vi "Find frequency.vi"() -> ()   [LabVIEW 2017]
uses:
  <vilib>/DAQmx/create/channels.llb/DAQmx Create Channel (AI-Voltage-Basic).vi
  <vilib>/measure/NI_MAPro.lvlib
  <vilib>/measure/madcrms.llb/Basic Averaged DC-RMS for 1 Chan.vi
  <vilib>/DAQmx/configure/timing.llb/DAQmx Timing (Sample Clock).vi
  <vilib>/DAQmx/read.llb/DAQmx Read (Analog 2D DBL NChan NSamp).vi
panel:
  in  "Delay, ms":u32=300
  out "Result":dbl
  in  "btnStartStop":bool=TRUE caption="stop"
  out "CurrentFrequency":dbl
  out "CurrentPoint":i32
  out "XY Graph":cluster{dbl[], dbl[]}[](graph)
  in  "Maximum Value":dbl=10.0 format="%0.2f"
  in  "Minimum Value":dbl=-10.0 format="%0.2f"
  in  "Rate":dbl=1000.0 caption="Sample Rate (Hz)" format="%0.2f"
  in  "Samples per Channel":i32=1000
  in  "Physical Channel":tag="Dev2/ai0:1"
  in  "btnStartStopScanning":bool=TRUE caption="stop"
  in  "btnQuit":bool caption="stop"
  out "FrequencyPoints":i32=1000 caption="Frequency points"
  in  "FrequencyStep":dbl=1000.0 caption="Frequency step, Hz"
  in  "EndFrequency":dbl=10000.0 caption="End frequency, Hz" format="%.2p"
  in  "resource name":refnum<k15>="test"
  in  "start phase":dbl format="%.3f"
  in  "StartFrequency":dbl=1000.0 caption="Start frequency, Hz" format="%.2p"
  in  "dc offset":dbl=0.5 format="%.3f"
  in  "Amplitude":dbl=1.0 format="%.3f"
  in  "channel name (\"1\")":string="1"
  in  "WaveformType":i32(ring)=1 items=["Sine"=1, "Square"=2, "Ramp Up"=4, "Triangle"=3, "DC "=6, "Noise"=1001, "Pulse"=1002, "Ramp Down"=5, "Ramp"=1004]
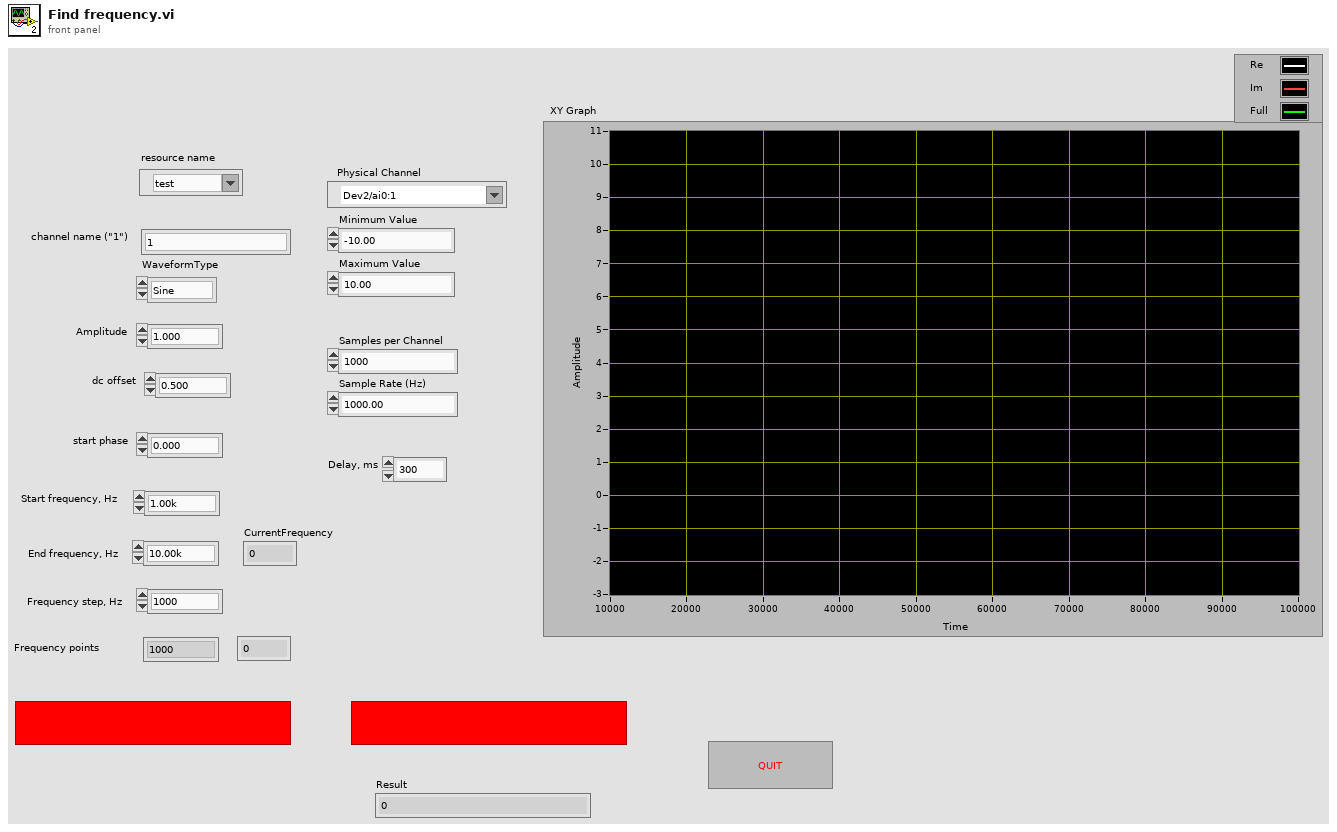
[diagram p1: front panel]
types:
  T1 = enum16{"Rectangular (none)", "Hanning", "Low side lobe"}
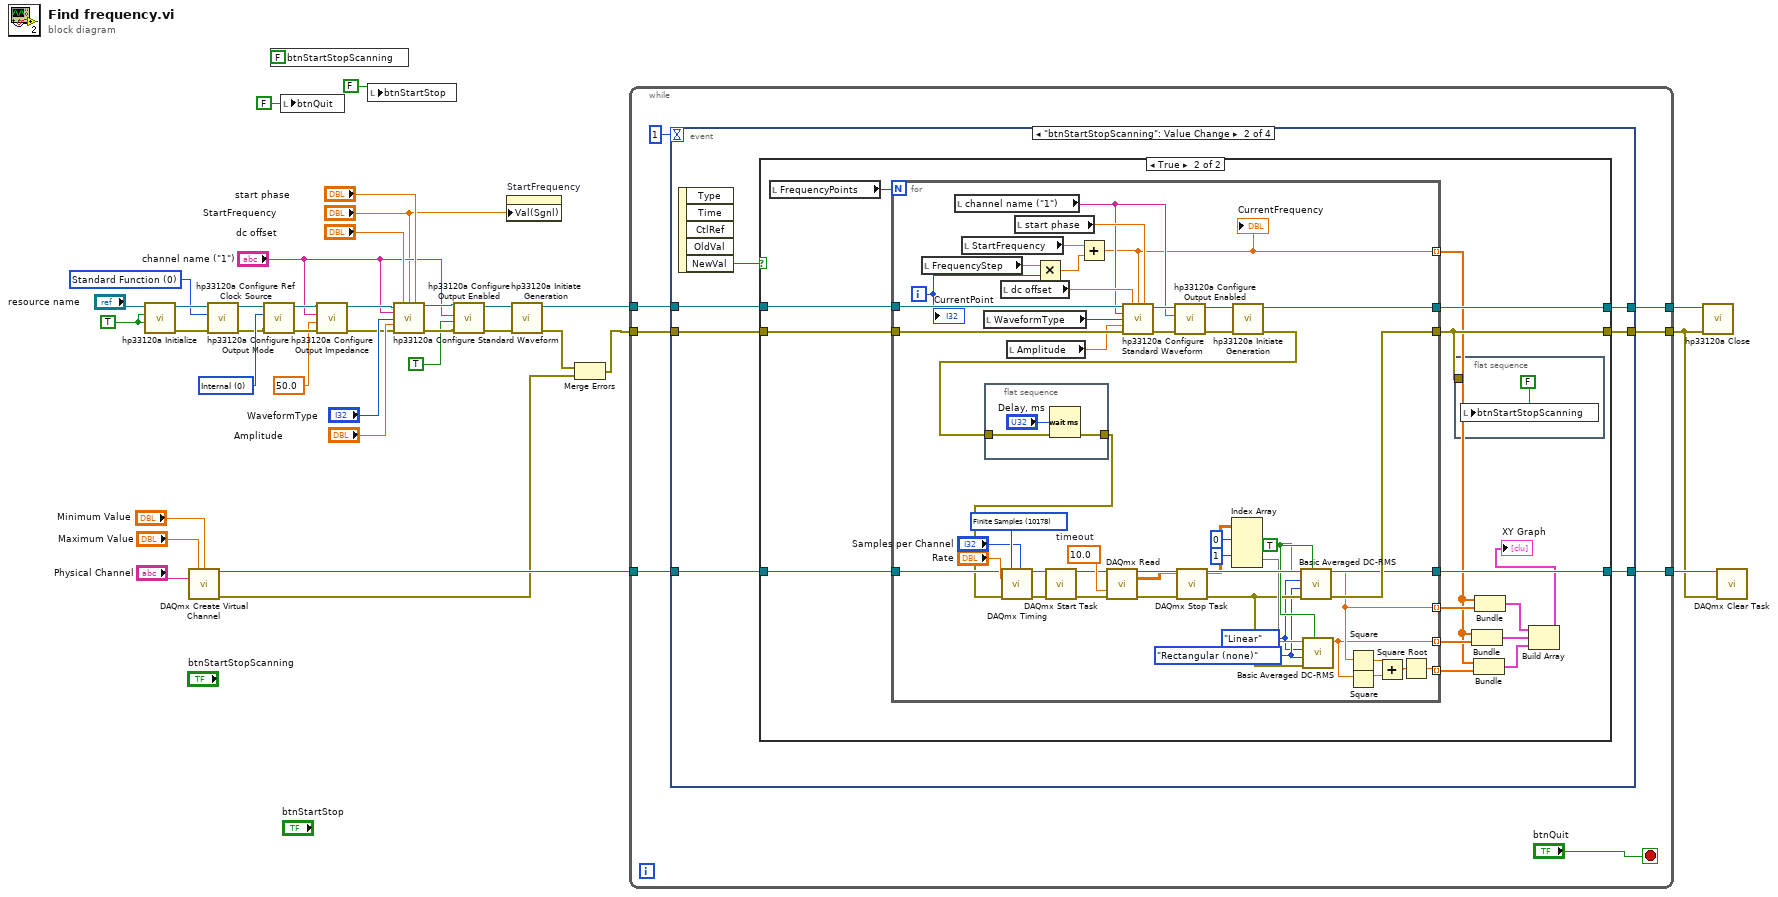
[diagram p0: block diagram]
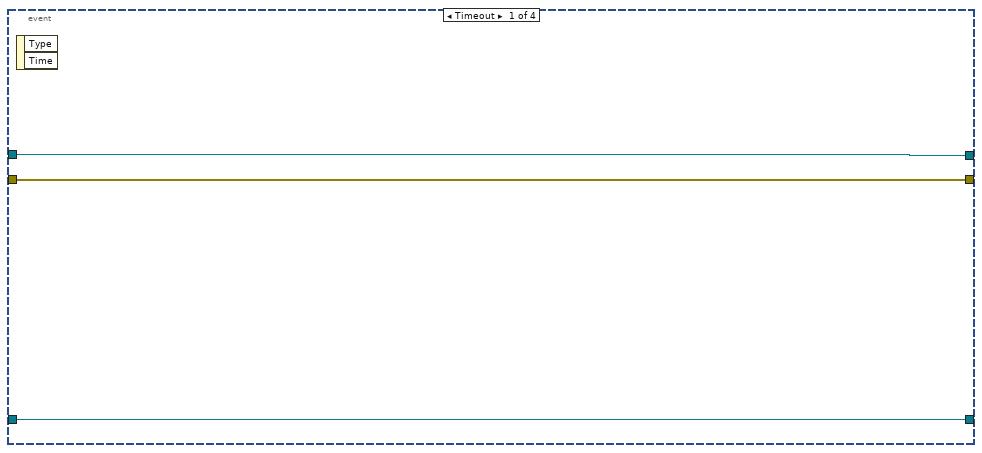
[diagram p2: hidden frame]
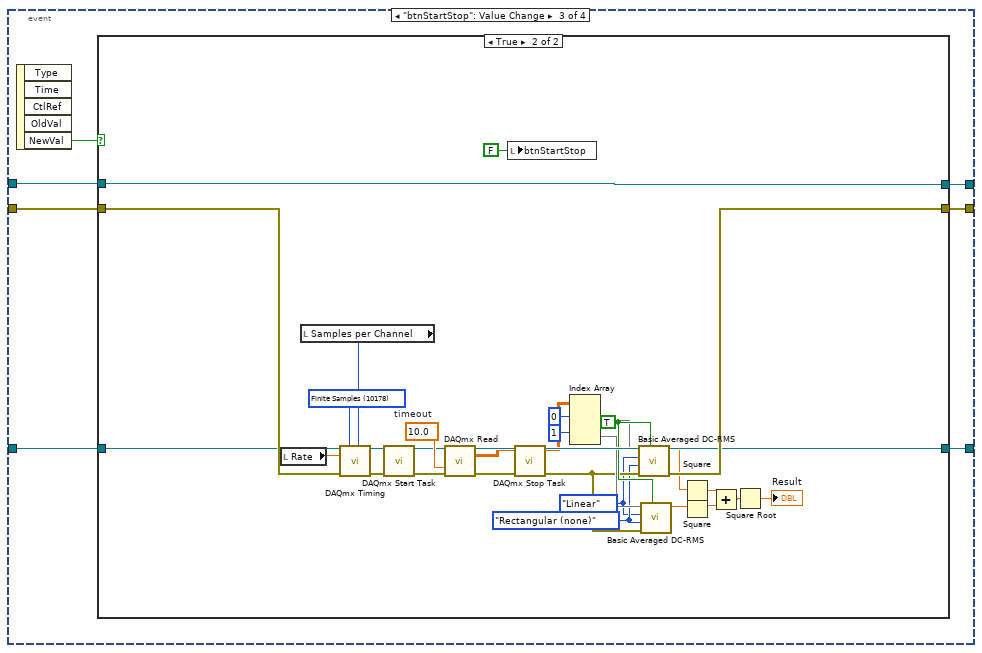
[diagram p4: hidden frame]
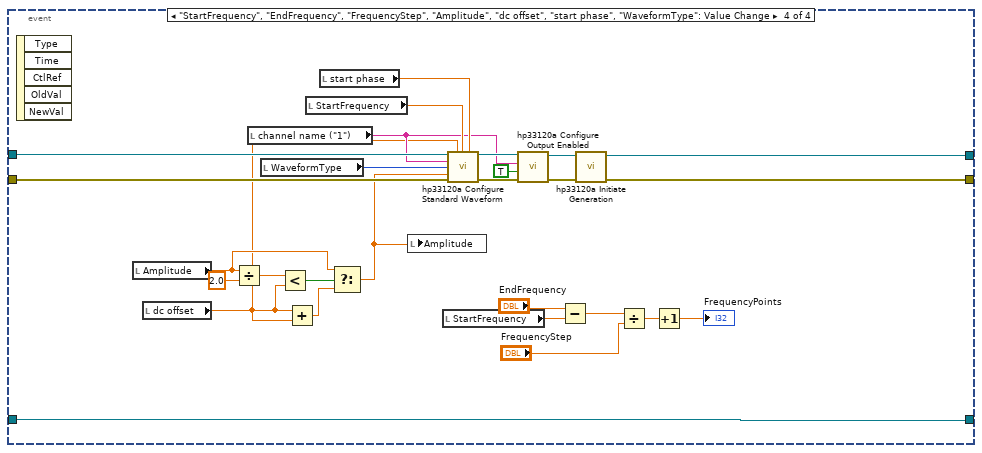
[diagram p6: hidden frame]
diagram:
  w33 = 0 items=["Internal"=0, "External"=1, "RTSI Clock"=101] ("reference clock source (Internal)")
  w34 = 0 items=["Standard Function", "Arbitrary Waveform", "Arbitrary Sequence"] ("output mode (Standard Function)")
  w37 = TRUE ("id query")
  n1 = call <instrlib>:"hp33120a Initialize.vi"("reset device (Yes)"=w37, "id query (Yes)"=w37, "resource name"="resource name") -> ("error out"=w35:errorcluster, "instrument handle out"=w36:refnum<k15>)  [unwired: 1 in, 6 out]
  n2 = call-poly <vilib>:"DAQmx Create Virtual Channel.vi"("maximum value"="Maximum Value", "minimum value"="Minimum Value", "physical channels"="Physical Channel") -> ("task out"=w4:refnum<k21>, "error out"=w3:errorcluster)  [unwired: 11 in]
  n3 = call <instrlib>:"hp33120a Configure Output Mode.vi"("error in (no error)"=w35, "output mode (Standard Function)"=w34, "instrument handle"=w36) -> ("error out"=w29:errorcluster, "instrument handle out"=w30:refnum<k15>)  [unwired: 7 out]
  n4 = call <instrlib>:"hp33120a Configure Ref Clock Source.vi"("error in (no error)"=w29, "reference clock source (Internal)"=w33, "instrument handle"=w30) -> ("error out"=w38:errorcluster, "instrument handle out"=w28:refnum<k15>)  [unwired: 7 out]
  n5 = local write "btnStartStopScanning"(FALSE ("btnStartStop")) -> ()
  n6 = local write "btnQuit"(FALSE ("btnQuit")) -> ()
  n7 = call <instrlib>:"hp33120a Configure Output Impedance.vi"("error in (no error)"=w38, "impedance (50.0)"=50.0 ("impedance (50 Ohms)"), "channel name (\"1\")"="channel name (\"1\")", "instrument handle"=w28) -> ("error out"=w20:errorcluster, "instrument handle out"=w21:refnum<k15>)  [unwired: 6 out]
  n8 = local write "btnStartStop"(FALSE ("btnStartStop")) -> ()
  n9 = call <instrlib>:"hp33120a Configure Standard Waveform.vi"("instrument handle"=w21, "dc offset (0.00)"="dc offset", "frequency (1000.0)"="StartFrequency", "start phase (0.00)"="start phase", "channel name (\"1\")"="channel name (\"1\")", "waveform (Sine)"="WaveformType", "amplitude (0.10)"="Amplitude", "error in (no error)"=w20) -> ("instrument handle out"=w19:refnum<k15>, "error out"=w18:errorcluster)  [unwired: 6 out]
  n10 = call <instrlib>:"hp33120a Configure Output Enabled.vi"("error in (no error)"=w18, "channel enabled (True)"=TRUE, "channel name (\"1\")"="channel name (\"1\")", "instrument handle"=w19) -> ("error out"=w16:errorcluster, "instrument handle out"=w17:refnum<k15>)  [unwired: 6 out]
  n11 = property on="StartFrequency" class="DigNum (strict)"("Val(Sgnl)"="StartFrequency") -> ()  [unwired: 2 in, 2 out]
  n12 = call <instrlib>:"hp33120a Initiate Generation.vi"("error in (no error)"=w16, "instrument handle"=w17) -> ("error out"=w7:errorcluster, "instrument handle out"=w23:refnum<k15>)  [unwired: 8 out]
  n13 = Merge Errors(w7, w3) -> (w6:errorcluster)
  n14 = while {
    tunnel: w23 -> [w46]
    tunnel: w6 -> [w45]
    tunnel: [w44] -> w22
    tunnel: [w43] -> w5
    tunnel: w4 -> [w41]
    tunnel: [w40] -> w8
    stop <- "btnQuit" stop-if-true
    n15 = event shown="[1] \"btnStartStopScanning\": Value Change" {
      selector: _ -> [_ _ _ _]
      dyn-events: _ -> [_ _ _ _]
      timeout: 1 -> [_ _ _ _]
      tunnel: w46 -> [w48 w56 w131 w189]
      tunnel: w45 -> [w49 w55 w130 w188]
      tunnel: [w48 w54 w129 w180] -> w44
      tunnel: [w49 w53 w128 w179] -> w43
      tunnel: w41 -> [w47 w51 w126 w169]
      tunnel: [w47 w50 w125 w169] -> w40
      event Timeout {
        n16 = event-data() -> ()  [unwired: 1 in, 2 out]
      }
      event "btnStartStopScanning": Value Change {
        n17 = event-data() -> ("NewVal"=w52:bool)  [unwired: 1 in, 4 out]
        n18 = case shown="True" w52 {
          tunnel: w56 -> [w58 w74]
          tunnel: w55 -> [w59 w73]
          tunnel: [w58 w72] -> w54
          tunnel: [w59 w70] -> w53
          tunnel: w51 -> [w57 w69]
          tunnel: [w57 w68] -> w50
          frame False {
          }
          frame True {
            n19 = local read "FrequencyPoints"() -> (w71:i32)
            n20 = for {
              N: w71 -> [_]
              tunnel: w74 -> [w121]
              tunnel: w73 -> [w122]
              tunnel: [w115] -> w72
              tunnel: [w103] -> w70
              tunnel: w69 -> [w97]
              tunnel: [w91] -> w68
              tunnel: [w104] -> w61 mode=indexing
              tunnel: [w81] -> w66 mode=indexing
              tunnel: [w80] -> w63 mode=indexing
              tunnel: [w76] -> w62 mode=indexing
              i -> [w113]
              w100 = 10178 items=["Finite Samples"=10178, "Continuous Samples"=10123] ("sample mode")
              w83 = T1."Rectangular (none)" ("window")
              w82 = enum16{"Linear", "Exponential"}."Linear" ("averaging type")
              w90 = TRUE ("reset")
              w106 = 10.0  # timeout
              n21 = local read "FrequencyStep"() -> (w114:dbl)
              n22 = local read "channel name (\"1\")"() -> (w109:string)
              n23 = local read "StartFrequency"() -> (w111:dbl)
              n24 = local read "WaveformType"() -> (w108:i32)
              n25 = flat-sequence {
                tunnel: w105 -> [w123]
                tunnel: [w123] -> w94
                frame #0 {
                  n26 = Wait (ms)(milliseconds to wait="Delay, ms") -> ()  [unwired: 1 out]
                }
              }
              n27 = local read "dc offset"() -> (w110:dbl)
              n28 = call-poly <vilib>:"DAQmx Timing.vi"("task/channels in"=w97, "sample mode"=w100, "samples per channel"="Samples per Channel", "rate"="Rate", "error in"=w94) -> ("task out"=w101:refnum<k21>, "error out"=w102:errorcluster)  [unwired: 9 in]
              n29 = local read "Amplitude"() -> (w107:dbl)
              n30 = local read "start phase"() -> (w120:dbl)
              n31 = Multiply(x=w114, y=w113) -> (x*y=w112:dbl)
              n32 = call <vilib>:"DAQmx Start Task.vi"("task/channels in"=w101, "error in"=w102) -> ("task out"=w96:refnum<k21>, "error out"=w95:errorcluster)  [unwired: 12 in]
              n33 = Add(x=w111, y=w112) -> (x+y=w104:dbl)
              "CurrentFrequency" <- w104
              n34 = call-poly <vilib>:"DAQmx Read.vi"("task/channels in"=w96, "timeout"=w106, "error in"=w95) -> ("task out"=w92:refnum<k21>, "data"=w89:dbl[][], "error out"=w93:errorcluster)  [unwired: 10 in]
              n35 = call <instrlib>:"hp33120a Configure Standard Waveform.vi"("instrument handle"=w121, "dc offset (0.00)"=w110, "frequency (1000.0)"=w104, "start phase (0.00)"=w120, "channel name (\"1\")"=w109, "waveform (Sine)"=w108, "amplitude (0.10)"=w107, "error in (no error)"=w122) -> ("instrument handle out"=w116:refnum<k15>, "error out"=w117:errorcluster)  [unwired: 6 out]
              n36 = call <instrlib>:"hp33120a Configure Output Enabled.vi"("error in (no error)"=w117, "channel name (\"1\")"=w109, "instrument handle"=w116) -> ("error out"=w118:errorcluster, "instrument handle out"=w119:refnum<k15>)  [unwired: 1 in, 6 out]
              n37 = call <vilib>:"DAQmx Stop Task.vi"("task/channels in"=w92, "error in"=w93) -> ("task out"=w91:refnum<k21>, "error out"=w84:errorcluster)  [unwired: 12 in]
              n38 = Index Array(array=w89, index (row) #1=0 ("index (row)"), index (row) #2=1 ("index (row)")) -> (element #1=w86:dbl[], element #2=w85:dbl[])  [unwired: 2 in]
              n39 = call <instrlib>:"hp33120a Initiate Generation.vi"("error in (no error)"=w118, "instrument handle"=w119) -> ("error out"=w105:errorcluster, "instrument handle out"=w115:refnum<k15>)  [unwired: 8 out]
              n40 = call-poly <vilib>:"Basic Averaged DC-RMS.vi"("reset"=w90, "error in (no error)"=w84, "window"=w83, "averaging type"=w82, "signal in"=w86) -> ("error out"=w103:errorcluster, "DC value"=w81:dbl)  [unwired: 3 in, 2 out]
              n41 = call-poly <vilib>:"Basic Averaged DC-RMS.vi"("reset"=w90, "error in (no error)"=w84, "window"=w83, "averaging type"=w82, "signal in"=w85) -> ("DC value"=w80:dbl)  [unwired: 3 in, 3 out]
              n42 = Square(x=w81) -> (x^2=w79:dbl)
              n43 = Square(x=w80) -> (x^2=w78:dbl)
              n44 = Add(x=w79, y=w78) -> (x+y=w77:dbl)
              n45 = Square Root(x=w77) -> (sqrt(x)=w76:dbl)
              "CurrentPoint" <- w113
            }
            n46 = flat-sequence {
              tunnel: w70 -> [_]
              frame #0 {
                n47 = local write "btnStartStopScanning"(FALSE ("btnStartStop")) -> ()
              }
            }
            n48 = Bundle(w61, w63) -> (w64:cluster{dbl[], dbl[]})  [unwired: 1 in]
            n49 = Bundle(w61, w62) -> (w60:cluster{dbl[], dbl[]})  [unwired: 1 in]
            n50 = Bundle(w61, w66) -> (w65:cluster{dbl[], dbl[]})  [unwired: 1 in]
            n51 = Build Array(w65, w64, w60) -> (→"XY Graph":cluster{dbl[], dbl[]}[])
          }
        }
      }
      event "btnStartStop": Value Change {
        n52 = event-data() -> ("NewVal"=w127:bool)  [unwired: 1 in, 4 out]
        n53 = case shown="True" w127 {
          tunnel: w131 -> [w133 w164]
          tunnel: w130 -> [w134 w165]
          tunnel: [w133 w164] -> w129
          tunnel: [w134 w163] -> w128
          tunnel: w126 -> [w132 w162]
          tunnel: [w132 w161] -> w125
          frame False {
          }
          frame True {
            w157 = 10178 items=["Finite Samples"=10178, "Continuous Samples"=10123] ("sample mode")
            w145 = T1."Rectangular (none)" ("window")
            w144 = enum16{"Linear", "Exponential"}."Linear" ("averaging type")
            w152 = TRUE ("reset")
            w160 = 10.0  # timeout
            n54 = local read "Rate"() -> (w136:dbl)
            n55 = local read "Samples per Channel"() -> (w137:i32)
            n56 = call-poly <vilib>:"DAQmx Timing.vi"("task/channels in"=w162, "sample mode"=w157, "samples per channel"=w137, "rate"=w136, "error in"=w165) -> ("task out"=w158:refnum<k21>, "error out"=w159:errorcluster)  [unwired: 9 in]
            n57 = call <vilib>:"DAQmx Start Task.vi"("task/channels in"=w158, "error in"=w159) -> ("task out"=w156:refnum<k21>, "error out"=w155:errorcluster)  [unwired: 12 in]
            n58 = call-poly <vilib>:"DAQmx Read.vi"("task/channels in"=w156, "timeout"=w160, "error in"=w155) -> ("task out"=w153:refnum<k21>, "data"=w151:dbl[][], "error out"=w154:errorcluster)  [unwired: 10 in]
            n59 = local write "btnStartStop"(FALSE ("btnStartStop")) -> ()
            n60 = call <vilib>:"DAQmx Stop Task.vi"("task/channels in"=w153, "error in"=w154) -> ("task out"=w161:refnum<k21>, "error out"=w146:errorcluster)  [unwired: 12 in]
            n61 = Index Array(array=w151, index (row) #1=0 ("index (row)"), index (row) #2=1 ("index (row)")) -> (element #1=w148:dbl[], element #2=w147:dbl[])  [unwired: 2 in]
            n62 = call-poly <vilib>:"Basic Averaged DC-RMS.vi"("reset"=w152, "error in (no error)"=w146, "window"=w145, "averaging type"=w144, "signal in"=w148) -> ("error out"=w163:errorcluster, "DC value"=w143:dbl)  [unwired: 3 in, 2 out]
            n63 = call-poly <vilib>:"Basic Averaged DC-RMS.vi"("reset"=w152, "error in (no error)"=w146, "window"=w145, "averaging type"=w144, "signal in"=w147) -> ("DC value"=w142:dbl)  [unwired: 3 in, 3 out]
            n64 = Square(x=w143) -> (x^2=w141:dbl)
            n65 = Square(x=w142) -> (x^2=w140:dbl)
            n66 = Add(x=w141, y=w140) -> (x+y=w139:dbl)
            n67 = Square Root(x=w139) -> (sqrt(x)=→"Result":dbl)
          }
        }
      }
      event "StartFrequency", "EndFrequency", "FrequencyStep", "Amplitude", "dc offset", "start phase", "WaveformType": Value Change {
        n68 = event-data() -> ()  [unwired: 1 in, 5 out]
        n69 = local read "Amplitude"() -> (w172:dbl)
        n70 = local read "dc offset"() -> (w171:dbl)
        n71 = Divide(x=w172, y=2.0) -> (x/y=w175:dbl)
        n72 = local read "channel name (\"1\")"() -> (w178:string)
        n73 = local read "WaveformType"() -> (w185:i32)
        n74 = Less?(x=w175, y=w171) -> (x < y?=w174:bool)
        n75 = Add(x=w171, y=w171) -> (x+y=w173:dbl)
        n76 = local read "StartFrequency"() -> (w186:dbl)
        n77 = local read "start phase"() -> (w187:dbl)
        n78 = Select(t=w172, s=w174, f=w173) -> (s? t:f=w170:dbl)
        n79 = local write "Amplitude"(w170) -> ()
        n80 = local read "StartFrequency"() -> (w191:dbl)
        n81 = call <instrlib>:"hp33120a Configure Standard Waveform.vi"("instrument handle"=w189, "dc offset (0.00)"=w171, "frequency (1000.0)"=w186, "start phase (0.00)"=w187, "channel name (\"1\")"=w178, "waveform (Sine)"=w185, "amplitude (0.10)"=w170, "error in (no error)"=w188) -> ("instrument handle out"=w181:refnum<k15>, "error out"=w182:errorcluster)  [unwired: 6 out]
        n82 = call <instrlib>:"hp33120a Configure Output Enabled.vi"("error in (no error)"=w182, "channel enabled (True)"=TRUE, "channel name (\"1\")"=w178, "instrument handle"=w181) -> ("error out"=w183:errorcluster, "instrument handle out"=w184:refnum<k15>)  [unwired: 6 out]
        n83 = Subtract(x="EndFrequency", y=w191) -> (x-y=w190:dbl)
        n84 = call <instrlib>:"hp33120a Initiate Generation.vi"("error in (no error)"=w183, "instrument handle"=w184) -> ("error out"=w179:errorcluster, "instrument handle out"=w180:refnum<k15>)  [unwired: 8 out]
        n85 = Divide(x=w190, y="FrequencyStep") -> (x/y=w167:dbl)
        n86 = Increment(x=w167) -> (x+1=→"FrequencyPoints":dbl)
      }
    }
  }
  n87 = call <instrlib>:"hp33120a Close.vi"("error in (no error)"=w5, "instrument handle"=w22) -> ()  [unwired: 10 out]
  n88 = call <vilib>:"DAQmx Clear Task.vi"("task in"=w8, "error in"=w5) -> ()  [unwired: 13 in, 1 out]
